vi "CAPFM-Init StimChans.vi"(0 "Params":T1, 2 "Data Folder":path, 11 "error in (no error)":errorcluster) -> (4 "StimChans":T8[](xcontrol), 15 "error out":errorcluster)   [LabVIEW 2020]
uses:
  epl-vi-lib/Signal Synthesis VIs/Controls/Stimulus Channel (Full)/Stimulus Channel (Full).xctl
  epl-vi-lib/Signal Synthesis VIs/Controls/Multichannel (Full)/Multichannel (Full).xctl
  Typedefs/CAPFM-All Params.ctl
  epl-vi-lib/Utility VIs/Type Defs/Left-Right ring.ctl
  Typedefs/CAPFM-Probe Params.ctl
  Typedefs/CAPFM-Masker Params.ctl
  Typedefs/CAPFM-Seq Params.ctl
  Typedefs/CAPFM-Timing Params.ctl
  Typedefs/CAPFM-Response Params.ctl
  epl-vi-lib/Signal Synthesis VIs/Controls/Waveform XCtl/Waveform Enum.ctl
  epl-vi-lib/Signal Synthesis VIs/Controls/Level XCtl/Level Units.ctl
  epl-vi-lib/Utility VIs/Type Defs/Speaker ring.ctl
panel:
  in  "Dummy":T33(xcontrol)
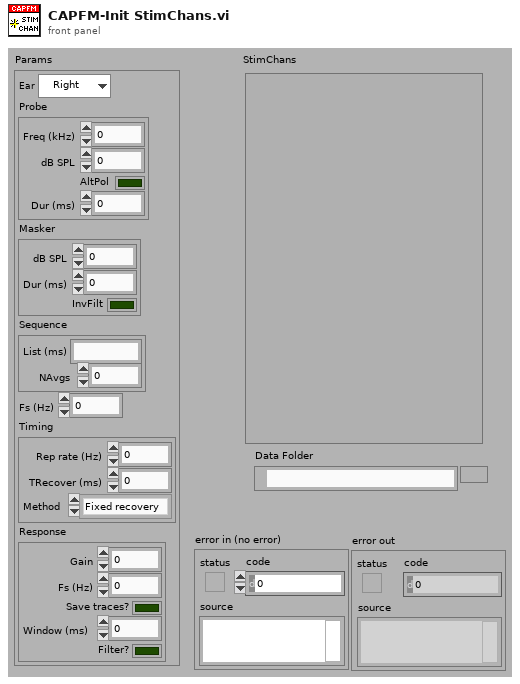
[diagram p1: front panel]
types:
  T1 = typedef "CAPFM-All Params.ctl" = cluster{"Ear":T2, "Probe":T3, "Masker":T4, "Sequence":T5, "Fs (Hz)":dbl, "Timing":T6, "Response":T7}
  T2 = typedef "Left-Right ring.ctl" = enum16{"Right", "Left"}
  T3 = typedef "CAPFM-Probe Params.ctl" = cluster{"Freq (kHz)":dbl, "dB SPL":dbl, "AltPol":bool, "Dur (ms)":dbl}
  T4 = typedef "CAPFM-Masker Params.ctl" = cluster{"dB SPL":dbl, "Dur (ms)":dbl, "InvFilt":bool}
  T5 = typedef "CAPFM-Seq Params.ctl" = cluster{"List (ms)":string, "NAvgs":i32}
  T6 = typedef "CAPFM-Timing Params.ctl" = cluster{"Rep rate (Hz)":dbl, "TRecover (ms)":dbl, "Method":enum16{"Fixed recovery", "Fixed rep rate"}}
  T7 = typedef "CAPFM-Response Params.ctl" = cluster{"Gain":dbl, "Fs (Hz)":dbl, "Save traces?":bool, "Window (ms)":dbl, "Filter?":bool}
  T8 = typedef "Stimulus Channel (Full).xctl/Full Stimulus Channel Data.ctl" = cluster{"Waveform":T9, "Filter":T26, "Burst":T28, "Level":T29, "Name":string, "Advanced":T31, "SAM":T32}
  T9 = typedef "Waveform XCtl.xctl/Waveform Data.ctl" = cluster{"Type":T10, "Tone":T11, "Pulse Train":T12, "Noise":T15, "File":T16, "FMSweep":T17, "Chirp Train":T18, "Complex Tone":cluster{"Params":T20, "Data":T22}, "Moving Ripple":T23}
  T10 = typedef "Waveform Enum.ctl" = enum16{"OFF", "Tone", "Noise", "Pulse Train", "File", "FM Sweep", "Chirp Train", "Complex Tone", "FM Tone", "Moving Ripple"}
  T11 = typedef "Tone Params.ctl" = cluster{"Frequency (kHz)":dbl, "Last Freq":dbl, "Last Phase":dbl}
  T12 = typedef "Pulse Train Params.ctl" = cluster{"Pulse width (us)":dbl, "Pulse rate (Hz)":dbl, "Gap (ms)":dbl, "Polarity":T13, "PT State":T14, "Asynch":bool}
  T13 = typedef "Pulse Polarity.ctl" = enum16{"POS", "NEG", "POS-NEG", "NEG-POS"}
  T14 = typedef "PT-Continuous State.ctl" = cluster{"Template":dbl[], "Nperiod":i32, "Index":i32, "Pulse Rate (Hz)":dbl, "Phase (cycles)":dbl, "Noff":i32}
  T15 = typedef "Noise Params.ctl" = cluster{"InvFilt":bool, "Noise":dbl[], "CurPt":i32, "Aweight":bool, "Seed":i32, "afile":path}
  T16 = typedef "StimFile-Params.ctl" = cluster{"Filename":path, "Signal":dbl[], "Channel":i32, "stream":bool, "offset":i32, "nreps":i32, "loops":i32, "Randomize":bool, "order":i32[], "Seed":i32, "Tokens":i32}
  T17 = typedef "FM Sweep Params.ctl" = cluster{"Rate (oct/s)":dbl, "Fmin (Hz)":dbl, "Fmax (Hz)":dbl, "Ramp (ms)":dbl, "Linear":bool}
  T18 = typedef "Chirp Train.ctl" = cluster{"Params":T19, "Data":cluster{"WF":dbl[]}}
  T19 = typedef "Chirp Train Params.ctl" = cluster{"Fmin (kHz)":dbl, "Fmax (kHz)":dbl, "Compensate":bool, "Duration (ms)":dbl}
  T20 = typedef "CT-Params.ctl" = cluster{"F0 (Hz)":dbl, "Band":cluster{"Flow (Hz)":dbl, "Fhigh (Hz)":dbl}, "Phase":T21, "Min F0 (Hz)":dbl, "Max F0 (Hz)":dbl, "ContinRandPhase":bool, "Max peak factor":dbl, "Max mod depth":dbl, "MinHarmNum":i32, "MaxHarmNum":i32, "Level Mode":enum16{"per component", "overall rms"}, "% jitter":dbl}
  T21 = typedef "CT-Phase Enum.ctl" = enum16{"Cosine", "Random", "Alternating"}
  T22 = typedef "CT-Runtime Data.ctl" = cluster{"Ncomp":i32, "MinHarm":i32, "Phase":dbl[], "Amplitude":dbl[], "Npts/frame":i32, "Last F0":dbl, "Fmin":dbl, "Fmax":dbl, "Lslope":dbl, "randphase":bool, "overall rms":bool, "fmult":dbl[], "jittered":bool}
  T23 = typedef "Moving Ripple.ctl" = cluster{"Params":T24, "Data":T25}
  T24 = typedef "Moving Ripple.Params.ctl" = cluster{"Fmin":dbl, "Fmax":dbl, "Density":dbl, "Velocity":dbl, "Depth":dbl, "Phase":dbl, "Comp/oct":i32}
  T25 = typedef "Moving Ripple.Data.ctl" = cluster{"Freq":dbl[], "A":dbl[], "phase":dbl[], "Phase":dbl}
  T26 = typedef "Advanced Filter XCtl.xctl/Filter Data.ctl" = cluster{"Type":enum16{"Lowpass", "Highpass", "Bandpass", "Bandstop", "OFF"}, "CF (kHz)":dbl, "BW (kHz)":dbl, "Cascade":bool, "Quadrature":bool, "Scale Factor":dbl, "Stages":cluster{"IIR Filter":cluster{"filter structure":enum32{"IIR 2nd Order", "IIR 4th Order"}, "Reverse Coefficients":dbl[], "Forward Coefficients":dbl[]}, "State":dbl[]}[], "Class":enum16{"Elliptic", "Butterworth"}, "Order":i32, "BWUnits":T27}
  T27 = typedef "Filter-Bandwidth Units.ctl" = enum16{"Linear", "Octaves", "Min-Max"}
  T28 = typedef "Burst Control.xctl/Burst Data.ctl" = cluster{"Active":bool, "Delay (ms)":dbl, "Duration (ms)":dbl, "Ramp (ms)":dbl, "Rate (Hz)":dbl, "Trepeat (ms)":dbl, "Repeat":bool}
  T29 = typedef "Level XCtl.xctl/Level Data.ctl" = cluster{"Level":dbl, "Units":T30, "Max":dbl, "Multiplier":dbl, "Cal File":path, "Cal":cluster{"Freq (Hz)":dbl[], "Mag (dB SPL)":dbl[], "Phase (deg)":dbl[]}}
  T30 = typedef "Level Units.ctl" = enum16{"dB atten", "dB SPL", "dB re 1 Vrms", "dB V/Hz½", "mW", "dB HL", "Volts", "dB mW"}
  T31 = typedef "Advanced Stimulus Options.xctl/Advanced Stimulus Options.ctl" = cluster{"Rep Mask":string, "AltPol":bool, "Var":string, "Expr":string, "Persist":bool}
  T32 = typedef "SAM Params.ctl" = cluster{"Active":bool, "Frequency (Hz)":dbl, "Depth":dbl, "Init Phase (cycles)":dbl, "phase (degrees)":dbl, "Asynch":bool}
  T33 = cluster{"Waveform":T9, "Filter":T26, "Burst":T28, "Level":T29, "Name":string, "Advanced":T31, "SAM":T32}
  T34 = enum16{"Lowpass", "Highpass", "Bandpass", "Bandstop", "OFF"}
  T35 = typedef "Speaker ring.ctl" = enum16{"Right primary", "Right secondary", "Left primary", "Left secondary"}
  T36 = cluster{"Waveform":T9, "Filter":T26, "Burst":T28, "Level":T29, "Name":string, "Advanced":T31, "SAM":T32}[]
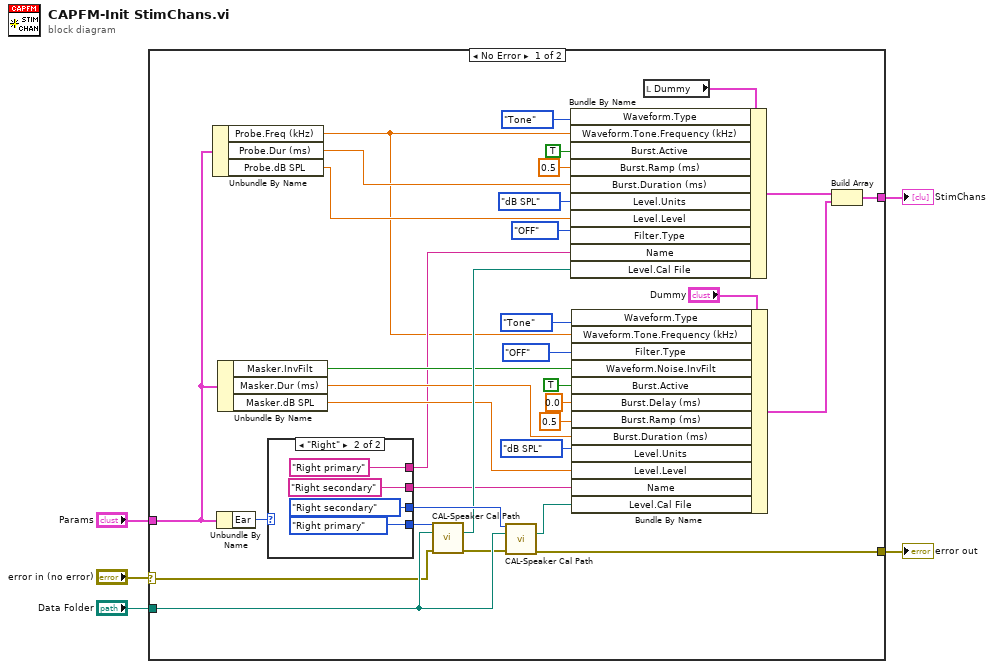
[diagram p0: block diagram]
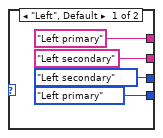
[diagram p2: hidden frame]
diagram:
  n1 = case shown="No Error" "error in (no error)" {
    selector: "error in (no error)" -> [w27 w48]
    tunnel: [w35 _] -> w5
    tunnel: "Params" -> [w15 _]
    tunnel: "Data Folder" -> [w33 _]
    tunnel: [w26 w48] -> w2
    frame No Error {
      n2 = Unbundle By Name(w15) -> ("Probe.Freq (kHz)"=w6:dbl, "Probe.Dur (ms)"=w12:dbl, "Probe.dB SPL"=w11:dbl)
      n3 = Unbundle By Name(w15) -> ("Ear"=w30:T2)
      n4 = Unbundle By Name(w15) -> ("Masker.InvFilt"=w23:bool, "Masker.Dur (ms)"=w19:dbl, "Masker.dB SPL"=w17:dbl)
      n5 = case shown="\"Right\"" w30 {
        tunnel: [Speaker_ring."Left primary" ("Speaker") Speaker_ring."Right primary" ("Speaker")] -> w34
        tunnel: [Speaker_ring."Left secondary" ("Speaker") Speaker_ring."Right secondary" ("Speaker")] -> w32
        tunnel: ["Left primary" "Right primary"] -> w9
        tunnel: ["Left secondary" "Right secondary"] -> w8
        frame "Left", Default {
        }
        frame "Right" {
        }
      }
      n6 = call "CAL-Speaker Cal Path.vi"("Speaker"=w34, "Data Folder"=w33, "error in (no error)"=w27) -> ("Cal Path"=w29:path, "error out"=w31:errorcluster)  [unwired: 11 in]
      n7 = call "CAL-Speaker Cal Path.vi"("Speaker"=w32, "Data Folder"=w33, "error in (no error)"=w31) -> ("Cal Path"=w28:path, "error out"=w26:errorcluster)  [unwired: 11 in]
      n8 = Bundle By Name(cluster="Dummy", "Waveform.Type"=Waveform_Enum."Tone" ("t"), "Waveform.Tone.Frequency (kHz)"=w6, "Filter.Type"=T34."OFF", "Waveform.Noise.InvFilt"=w23, "Burst.Active"=TRUE, "Burst.Delay (ms)"=0.0, "Burst.Ramp (ms)"=0.5, "Burst.Duration (ms)"=w19, "Level.Units"=Level_Units."dB SPL" ("Level.Mode"), "Level.Level"=w17, "Name"=w8, "Level.Cal File"=w28) -> (w36:T33)
      n9 = local read "Dummy"() -> (w25:T33)
      n10 = Bundle By Name(cluster=w25, "Waveform.Type"=Waveform_Enum."Tone", "Waveform.Tone.Frequency (kHz)"=w6, "Burst.Active"=TRUE, "Burst.Ramp (ms)"=0.5, "Burst.Duration (ms)"=w12, "Level.Units"=Level_Units."dB SPL" ("Level.Mode"), "Level.Level"=w11, "Filter.Type"=T34."OFF", "Name"=w9, "Level.Cal File"=w29) -> (w10:T33)
      n11 = Build Array(w10, w36) -> (w35:T36)
    }
    frame Error {
    }
  }
  "error out" <- w2
  "StimChans" <- w5
